vi "Hex File Path.vi"(0 "Device Reference in":T1 format="%.0x", 11 "error in (no error)":errorcluster) -> (4 "Device Reference out":T1 format="%.0x", 6 "appended path":path, 15 "error out":errorcluster)   [LabVIEW 2014, in "AIT 664 Custom Device.lvlib"]
doc: "Given the device refeference find the HEX file path in Windows and RT depending on OS."
uses:
  AIT 664 Custom Device.lvlib
  <vilib>/NI Veristand/Custom Device API/Custom Device Item Ref.ctl
  <vilib>/NI Veristand/Custom Device API/Get Item Property (Boolean).vi
  Controls and Global/Global.vi
  <vilib>/NI Veristand/Custom Device API/Get Item Property (Path).vi
  <vilib>/NI Veristand/Custom Device API/Custom Device API.lvlib
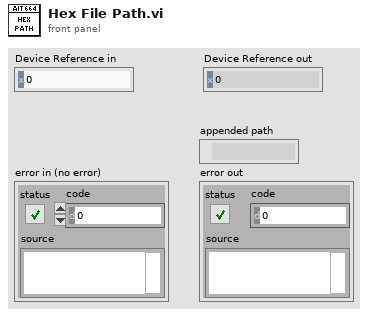
[diagram p1: front panel]
types:
  T1 = typedef "Custom Device API.lvlib/Custom Device Item Ref.ctl" = u64
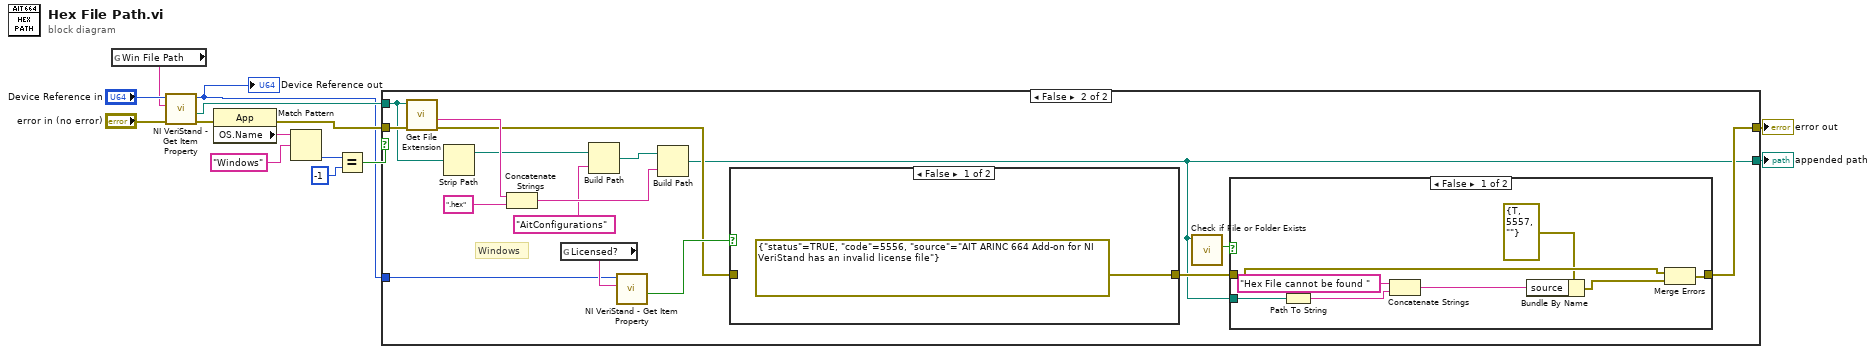
[diagram p0: block diagram]
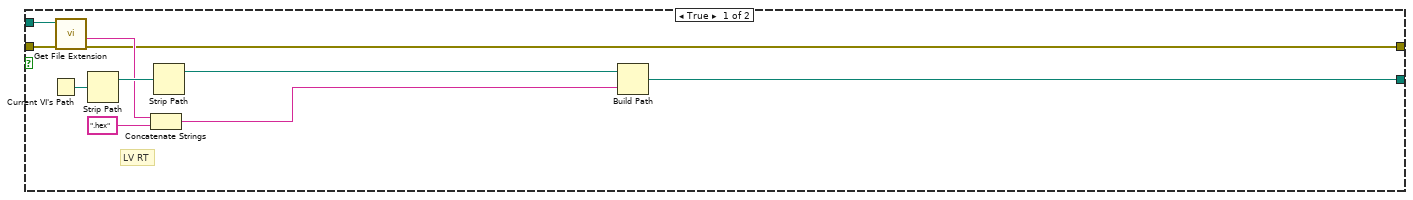
[diagram p2: hidden frame]
diagram:
  n1 = global read "Global.vi" "Win File Path"() -> (w11:string)
  n2 = call-poly <vilib>:"NI VeriStand - Get Item Property.vi"("error in (no error)"="error in (no error)", "Property Name"=w11, "Item Ref in"="Device Reference in") -> ("error out"=w4:errorcluster, "Value"=w3:path, "Item Ref out"=w1:T1)  [unwired: 5 in, 1 out]
  "Device Reference out" <- w1
  n3 = property class="App"(error in=w4) -> (error out=w8:errorcluster, "OS.Name"=w10:string)  [unwired: 1 in, 1 out]
  n4 = Match Pattern(string=w10, regular expression="Windows") -> (offset past match=w6:i32)  [unwired: 1 in, 3 out]
  n5 = Equal?(x=w6, y=-1) -> (x = y?=w9:bool)
  n6 = case shown="False" w9 {
    tunnel: w8 -> [w15 w37]
    tunnel: w3 -> [w18 w36]
    tunnel: [w17 w26] -> w14
    tunnel: [w16 w25] -> w2
    tunnel: w1 -> [_ w31]
    frame True {
      # "LV RT"
      n7 = Current VI's Path() -> (path=w20:path)
      n8 = call <vilib>:"Get File Extension.vi"("error in (no error)"=w15, "file"=w18) -> ("error out"=w17:errorcluster, "filename without extension"=w19:string)  [unwired: 6 in, 2 out]
      n9 = Strip Path(path=w20) -> (stripped path=w21:path)  [unwired: 1 out]
      n10 = Concatenate Strings(w19, ".hex" ("string")) -> (w23:string)
      n11 = Strip Path(path=w21) -> (stripped path=w22:path)  [unwired: 1 out]
      n12 = Build Path(base path=w22, name or relative path=w23) -> (appended path=w16:path)
    }
    frame False {
      # "Windows"
      n13 = call <vilib>:"Get File Extension.vi"("error in (no error)"=w37, "file"=w36) -> ("error out"=w29:errorcluster, "filename without extension"=w38:string)  [unwired: 6 in, 2 out]
      n14 = Strip Path(path=w36) -> (stripped path=w34:path)  [unwired: 1 out]
      n15 = Concatenate Strings(w38, ".hex" ("string")) -> (w39:string)
      n16 = global read "Global.vi" "Licensed?"() -> (w32:string)
      n17 = Build Path(base path=w34, name or relative path="AitConfigurations") -> (appended path=w35:path)
      n18 = call-poly <vilib>:"NI VeriStand - Get Item Property.vi"("Property Name"=w32, "Item Ref in"=w31) -> ("Value"=w30:bool)  [unwired: 6 in, 3 out]
      n19 = Build Path(base path=w35, name or relative path=w39) -> (appended path=w25:path)
      n20 = case shown="False" w30 {
        tunnel: w29 -> [_ w51]
        tunnel: [errorcluster {"status"=TRUE, "code"=5556, "source"="AIT ARINC 664 Add-on for NI VeriStand has an invalid license file"} ("error out") w51] -> w28
        frame False {
        }
        frame True {
        }
      }
      n21 = call <vilib>:"Check if File or Folder Exists.vi"("path"=w25) -> ("file or folder exists?"=w27:bool)  [unwired: 8 in, 2 out]
      n22 = case shown="False" w27 {
        tunnel: w28 -> [w47 w49]
        tunnel: [w48 w49] -> w26
        tunnel: w25 -> [w45 _]
        frame False {
          n23 = Path To String(path=w45) -> (string=w44:string)
          n24 = Concatenate Strings("Hex File cannot be found " ("string"), w44) -> (w42:string)
          n25 = Bundle By Name(cluster=errorcluster {"status"=TRUE, "code"=5557, "source"=""} ("error out"), "source"=w42) -> (w41:errorcluster)
          n26 = Merge Errors(w47, w41) -> (w48:errorcluster)
        }
        frame True {
        }
      }
    }
  }
  "error out" <- w14
  "appended path" <- w2
